vi "45.vi"() -> ()   [LabVIEW 2021]
panel:
  out "Array":i32[](array[numeric])
  in  "Numeric":i32=100000
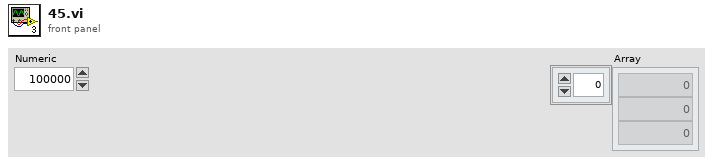
[diagram p1: front panel]
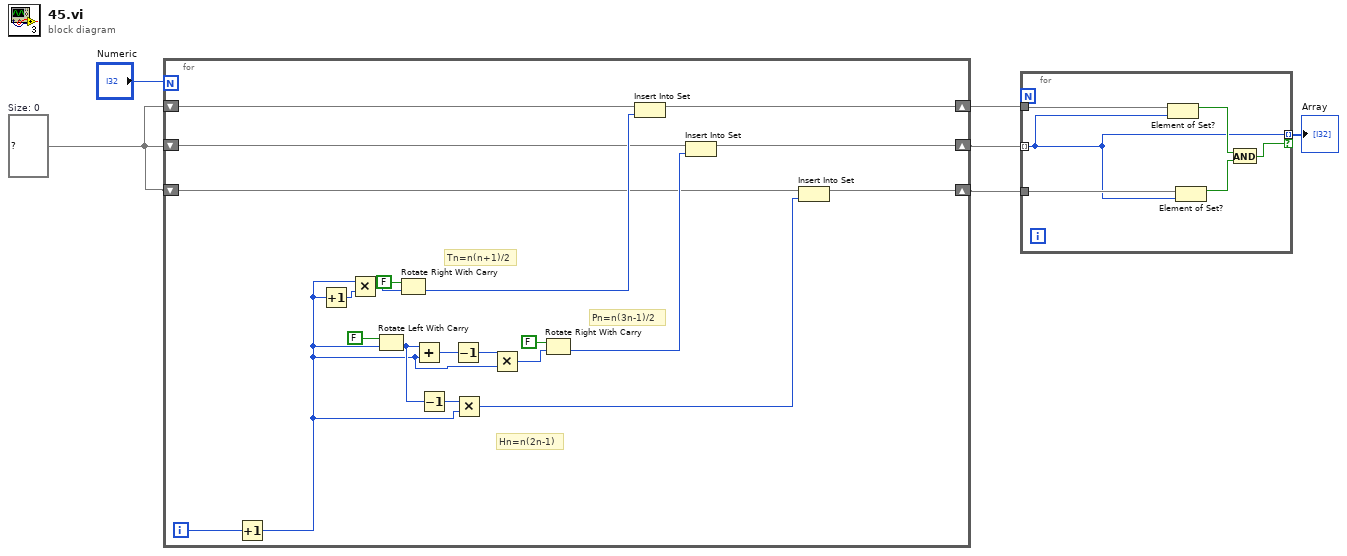
[diagram p0: block diagram]
diagram:
  w5 = set{i32} {}  # Size: 0
  n1 = for {
    N: "Numeric" -> [_]
    shift-right: [w14] -> w4
    shift-left: w5 -> [w15]
    shift-right: [w12] -> w3
    shift-left: w5 -> [w11]
    shift-right: [w9] -> w2
    shift-left: w5 -> [w7]
    i -> [w26]
    # "Hn=n(2n-1)"
    # "Pn=n(3n-1)/2"
    # "Tn=n(n+1)/2"
    n2 = Increment(x=w26) -> (x+1=w16:i32)
    n3 = Increment(x=w16) -> (x+1=w27:i32)
    n4 = Multiply(x=w16, y=w27) -> (x*y=w25:i32)
    n5 = Rotate Left With Carry(2:w16, 3:FALSE ("carry")) -> (0:w18:i32)  [unwired: 1 out]
    n6 = Rotate Right With Carry(2:w25, 3:FALSE ("carry")) -> (0:w13:i32)  [unwired: 1 out]
    n7 = Add(x=w18, y=w16) -> (x+y=w22:i32)
    n8 = Decrement(x=w18) -> (x-1=w17:i32)
    n9 = Decrement(x=w22) -> (x-1=w21:i32)
    n10 = Multiply(x=w17, y=w16) -> (x*y=w8:i32)
    n11 = Multiply(x=w21, y=w16) -> (x*y=w19:i32)
    n12 = Rotate Right With Carry(2:w19, 3:FALSE ("carry")) -> (0:w10:i32)  [unwired: 1 out]
    n13 = Insert Into Set(10:w13, 11:w15) -> (3:w14:set{i32})  [unwired: 1 out]
    n14 = Insert Into Set(10:w10, 11:w11) -> (3:w12:set{i32})  [unwired: 1 out]
    n15 = Insert Into Set(10:w8, 11:w7) -> (3:w9:set{i32})  [unwired: 1 out]
  }
  n16 = for {
    tunnel: w4 -> [w33]
    tunnel: w3 -> [w29] mode=indexing
    tunnel: w2 -> [w32]
    tunnel: [w29] -> w1 mode=indexing if=w28
    n17 = Element of Set?(10:w29, 11:w33) -> (3:w31:bool)
    n18 = Element of Set?(10:w29, 11:w32) -> (3:w30:bool)
    n19 = And(x=w31, y=w30) -> (x .and. y?=w28:bool)
  }
  "Array" <- w1
